vi "Write and Read.vi"(1 "Data":string, 2 "VISA resource name":refnum<visa-resource-name>="COM1", 3 "Addr (0-15)":i8 min=0 max=15 step=1) -> (0 "Write OK":bool)   [LabVIEW 2012]
doc: "The Basic Serial Read and Write example performs a Serial Port Read, a Serial Port Write, or a combination of these actions. The user selects the actions (read or write) on the front panel. If both are selected, the VI will write the data first, read data, and then close the VISA session that is opened to the port. This VI will wait until the specified number of bytes is received at the port or until a termination character is read.\n\nINSTRUCTIONS:\n1) Select the serial resource and configuration parameters (baud rate, data bits, parity, stop bits, flow control).\n2) Select the operations to be performed. \n3) Connect the serial port to your device. If no device is available, perform a loopback test by doing one of the following. Short pins 2 and 3 on a RS-232 cable or short pin 4 to pin 8 and pin 5 to pin 9 on a RS-485/422 cable. \n4) Run the VI to see the data read. (The \"read string\" will match the \"string to write\" if a loopback test was performed.)\n\nNote: The parameters set for the serial port must match the parameters of the connected instrument or device. In this example, the bytes to read parameter specifies the number of bytes that the serial port reads. If there were more bytes at the port than the number specified in bytes to read, those bytes would not be read. Also, if you specify to read more bytes than the number of bytes actually read, you might receive a timeout error message.\n\nOn the block diagram, the Configure Serial Port VI sets the configuration parameters. The front panel displays the controls used to configure the basic parameters, such as baud rate, data bits, and parity. Constants configure the other parameters the user probably does not need set. After the VISA Configure Serial Port VI opens the VISA session and configures the port, the VI passes the VISA resource name to other VIs that perform operations on that VISA resource. The VISA Write function sends a command to the serial device and the VISA Read function returns data based on the command. The VISA Close function then closes the reference to the serial device. It is important to close the reference; otherwise communication through with that port through protocols other than VISA might not be possible."
uses:
  <vilib>/Instr/_visa.llb/VISA Configure Serial Port (Instr).vi
panel:
  out "return count":u32
  in  "Length":u8=78
  in  "Offset":i16[](array[numeric])=[0, 0]
  in  "Write":bool=TRUE
  out "string to write":string="*IDN?\n"
  out "bytes read":u32
  out "read string":string
  # "Select the serial resource and the operations (Read, Write, or both) to be performed.  If both are selected, the VI will write the data first, read data and then close the VISA session that is opened to the port.  This VI will wait until the specified number of bytes is received at the port or until a termination character is read."
  # "For additional information select File >> VI Properties >> Documentation"
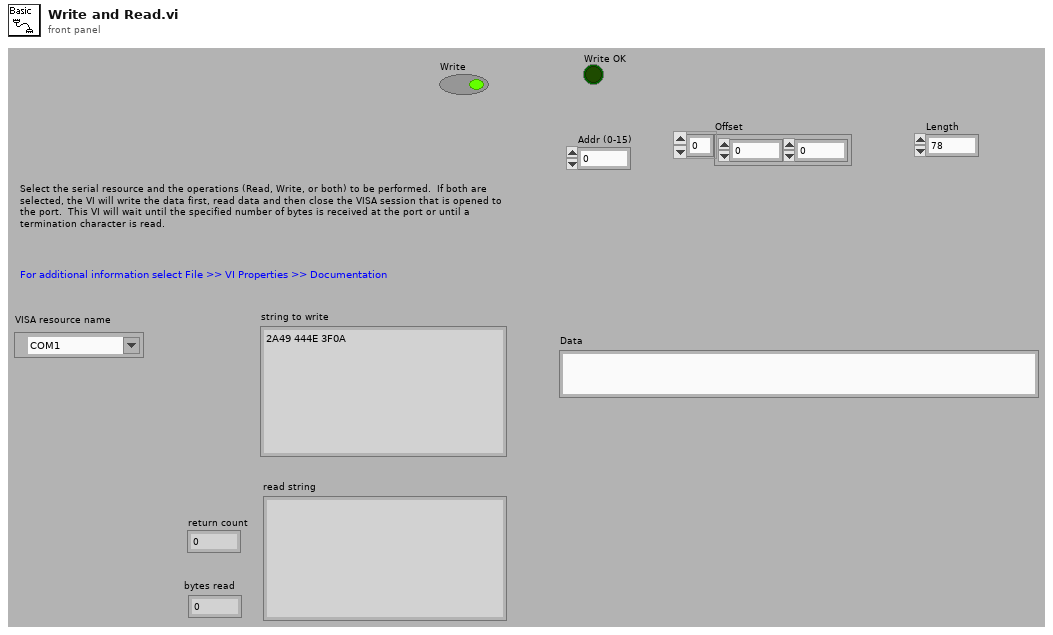
[diagram p1: front panel]
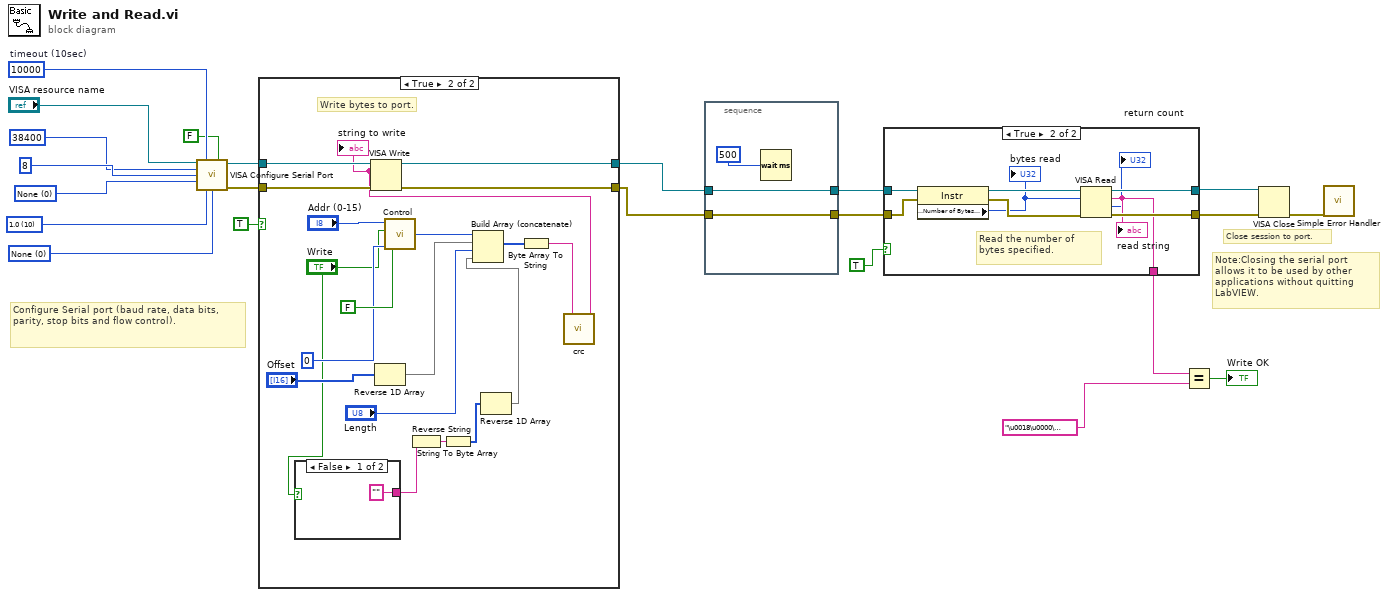
[diagram p0: block diagram]
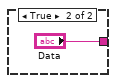
[diagram p3: hidden frame]
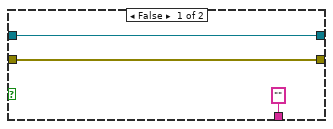
[diagram p4: hidden frame]
diagram:
  w12 = u16 0 items=["None"=0, "XON/XOFF"=1, "RTS/CTS"=2, "DTR/DSR"=4] ("flow control")
  w13 = u16 10 items=["1.0"=10, "1.5"=15, "2.0"=20] ("stop bits")
  w15 = u16 0 items=["None", "Odd", "Even", "Mark", "Space"] ("parity")
  w14 = u32 10000  # timeout (10sec)
  # "Note:Closing the serial port allows it to be used by other applications without quitting LabVIEW."
  # "Configure Serial port (baud rate, data bits, parity, stop bits and flow control)."
  # "Close session to port."
  n1 = call-poly "VISA Configure Serial Port"("VISA resource name"="VISA resource name", "timeout (10sec)"=w14, "Enable Termination\nChar (T)"=FALSE ("Enable Termination\nChar (T)"), "baud rate (9600)"=u32 38400, "data bits (8)"=u16 8 ("data bits"), "parity (0:none)"=w15, "stop bits (10: 1 bit)"=w13, "flow control (0:none)"=w12) -> ("VISA resource name out"=w19:refnum<visa-resource-name>, "error out"=w20:errorcluster)  [unwired: 1 in, 5 out]
  n2 = case shown="True" TRUE ("write") {
    tunnel: [w24 w43] -> w9
    tunnel: w19 -> [w23 w42]
    tunnel: w20 -> [w24 w41]
    tunnel: [w23 w40] -> w7
    frame False {
    }
    frame True {
      # "Write bytes to port."
      n3 = case shown="False" "Write" {
        tunnel: ["" ("Data") "Data"] -> w32
        frame False {
        }
        frame True {
        }
      }
      n4 = Reverse 1D Array(array="Offset") -> (reversed array=w34:i16[])
      n5 = call "Control.vi"("Page"=i8 0, "Error"=FALSE, "Write"="Write", "Addr"="Addr (0-15)") -> ("Control Byte"=w36:u32)
      n6 = Reverse String(1:w32) -> (0:w26:string)
      n7 = String To Byte Array(string=w26) -> (unsigned byte array=w31:u8[])
      n8 = Reverse 1D Array(array=w31) -> (reversed array=w30:u8[])
      n9 = Build Array (concatenate)(w36, w34, "Length", w30) -> (w29:u32[])
      n10 = Byte Array To String(unsigned byte array=w29) -> (string=w28:string)
      n11 = call "crc.vi"("Input string"=w28) -> ("Output (with crc)"=w27:string)
      "string to write" <- w27
      n12 = VISA Write(VISA resource name=w42, write buffer=w27, error in (no error)=w41) -> (VISA resource name out=w40:refnum<visa-resource-name>, error out=w43:errorcluster)  [unwired: 1 out]
    }
  }
  n13 = stacked-sequence {
    tunnel: w9 -> [w48]
    tunnel: [w48] -> w8
    tunnel: w7 -> [w47]
    tunnel: [w47] -> w6
    frame #0 {
      n14 = Wait (ms)(milliseconds to wait=u32 500 ("delay before read (ms)")) -> ()  [unwired: 1 out]
    }
  }
  n15 = case shown="True" TRUE ("read") {
    tunnel: w8 -> [w51 w56]
    tunnel: [w51 w60] -> w18
    tunnel: [w50 w59] -> w17
    tunnel: w6 -> [w50 w58]
    tunnel: ["" ("read buffer") w53] -> w4
    frame False {
    }
    frame True {
      # "Read the number of bytes specified."
      n16 = property class="Instr"(reference=w58, error in=w56) -> (reference out=w57:refnum<visa-resource-name>, error out=w55:errorcluster, "Serial Settings:Number of Bytes at Serial Port"=w54:u32)
      "bytes read" <- w54
      n17 = VISA Read(VISA resource name=w57, byte count=w54, error in (no error)=w55) -> (VISA resource name out=w59:refnum<visa-resource-name>, read buffer=w53:string, return count=→"return count":u32, error out=w60:errorcluster)
      "read string" <- w53
    }
  }
  n18 = Equal?(x=w4, y="\u0018\u0000\u0000N:") -> (x = y?=→"Write OK":bool)
  n19 = VISA Close(VISA resource name=w17, error in (no error)=w18) -> (error out=w16:errorcluster)
  n20 = call <vilib>:"Simple Error Handler.vi"("error in (no error)"=w16) -> ()  [unwired: 1 in, 8 out]
